vi "05 - Tip - Achieving Deterministic Handling Order.vi"() -> ()   [LabVIEW 2012]
panel:
  in  "Generate Events":enum16{"Greater than 1msec", "Sub-millisecond"}(ring)
  in  "Control":bool
  out "Static Event Registration":i32(graph)
  out "Dynamic Event Registration":i32(graph)
  out "Unique Event Queue":i32(graph)
  # "Conclusion:\nAll events within a single Events Queue will be handled deterministically;\nevents in separate Events Queues will be handled with millisecond accuracy,\nbut could become out of order with sub-millisecond resolution.\n\nBut don't count on handling order, especially near the 1msec threshold."
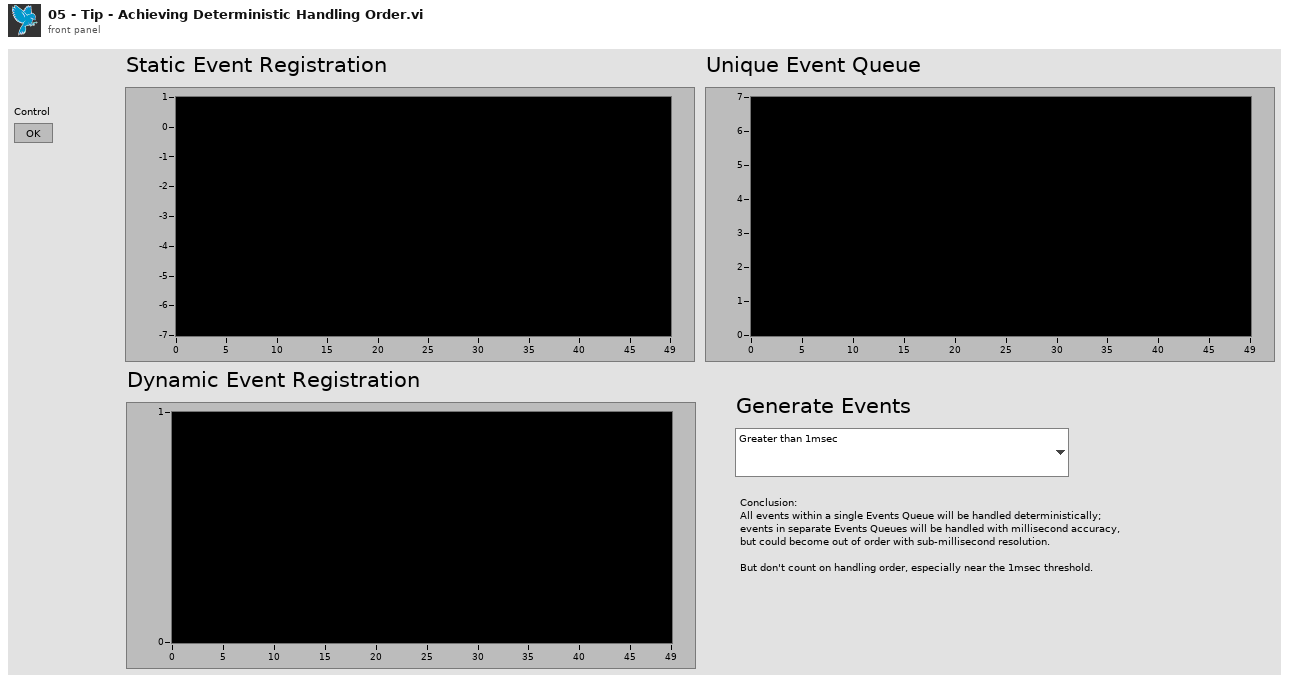
[diagram p1: front panel]
types:
  T1 = cluster{"Event Registration Refnum":refnum<event-registration>, "Event Registration Refnum":refnum<event-registration>}
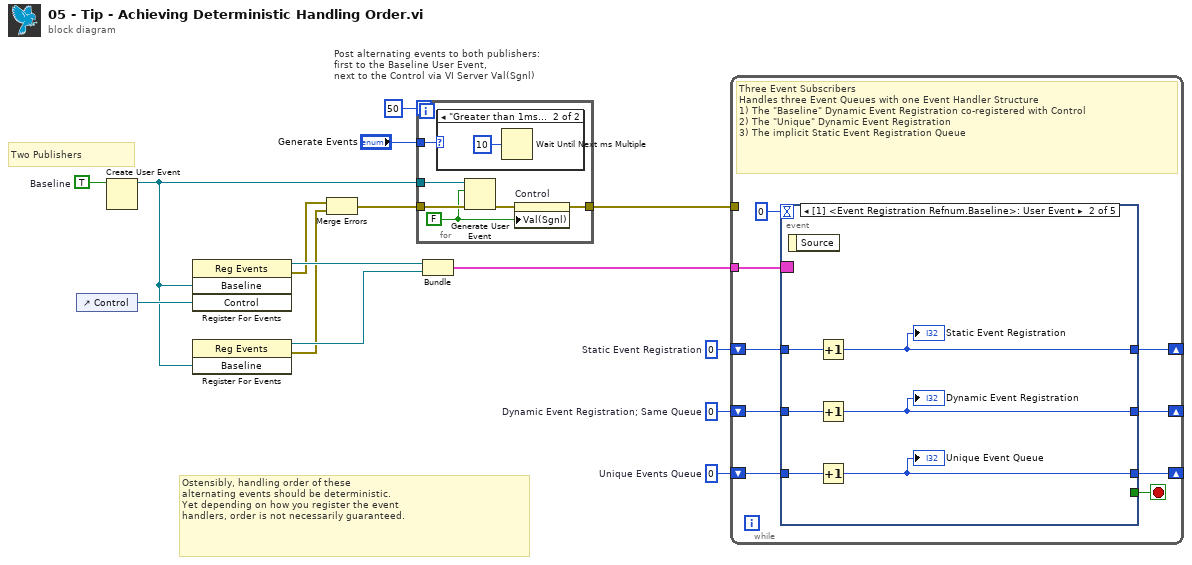
[diagram p0: block diagram]
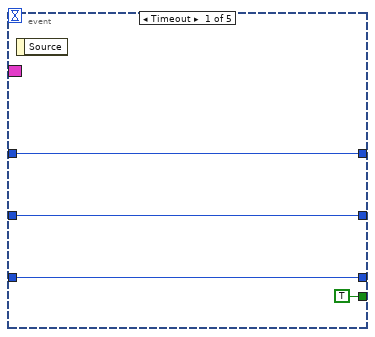
[diagram p3: hidden frame]
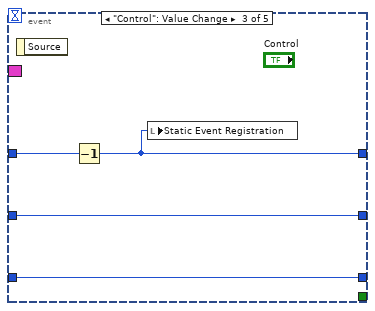
[diagram p4: hidden frame]
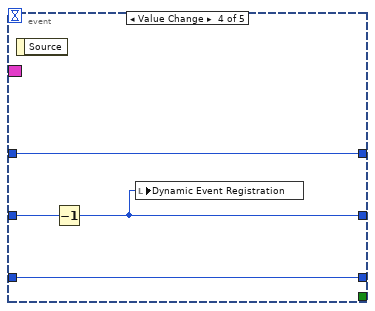
[diagram p5: hidden frame]
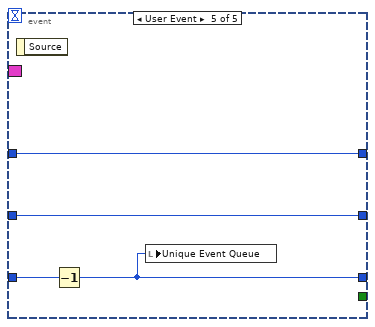
[diagram p6: hidden frame]
diagram:
  w5 = 0  # Unique Events Queue
  w10 = 0  # Dynamic Event Registration; Same Queue
  w12 = 0  # Static Event Registration
  w15 = TRUE  # Baseline
  # "Two Publishers"
  # "Ostensibly, handling order of these\nalternating events should be deterministic.\nYet depending on how you register the event\nhandlers, order is not necessarily guaranteed."
  n1 = control-ref of="Control"() -> (w11:refnum<vi>)
  n2 = Create User Event(user event datatype=w15) -> (user event=w9:refnum<user-event>)  [unwired: 1 in, 1 out]
  n3 = register-events(w9, w11) -> (reference out=w8:refnum<event-registration>, error out=w4:errorcluster)  [unwired: 2 in]
  n4 = register-events(w9) -> (reference out=w6:refnum<event-registration>, error out=w3:errorcluster)  [unwired: 2 in]
  n5 = Merge Errors(w4, w3) -> (w2:errorcluster)
  n6 = for "Post alternating events to both publishers:\nfirst to the Baseline User Event,\nnext to the Control via VI Server Val(Sgnl)" {
    N: 50 -> [_]
    tunnel: w9 -> [w20]
    tunnel: w2 -> [w19]
    tunnel: [w18] -> w13
    tunnel: "Generate Events" -> [w16]
    w17 = FALSE ("Value (Signaling)")
    n7 = case shown="\"Greater than 1msec\"" w16 {
      frame "Sub-millisecond" {
      }
      frame "Greater than 1msec" {
        n8 = Wait Until Next ms Multiple(millisecond multiple=u32 10 ("milliseconds to wait")) -> ()  [unwired: 1 out]
      }
    }
    n9 = Generate User Event(user event=w20, event data cluster=w17, error in=w19) -> (error out=w21:errorcluster)  [unwired: 1 out]
    n10 = property on="Control" class="Bool (strict)"(error in=w21, "Val(Sgnl)"=w17) -> (error out=w18:errorcluster)  [unwired: 1 in, 1 out]
  }
  n11 = Bundle("Event Registration Refnum"=w8, "Event Registration Refnum"=w6) -> (w7:T1)  [unwired: 1 in]
  n12 = while {
    tunnel: w7 -> [w31]
    tunnel: w13 -> [_]
    shift-right: [w27] -> _
    shift-left: w12 -> [w28]
    shift-right: [w25] -> _
    shift-left: w10 -> [w26]
    shift-right: [w24] -> _
    shift-left: w5 -> [w23]
    stop <- w30 stop-if-true
    # "Three Event Subscribers\nHandles three Event Queues with one Event Handler Structure\n1) The \"Baseline\" Dynamic Event Registration co-registered with Control\n2) The \"Unique\" Dynamic Event Registration\n3) The implicit Static Event Registration Queue"
    n13 = event shown="[1] <Event Registration Refnum.Baseline>: User Event" {
      selector: w31 -> [_ _ _ _ _]
      dyn-events: _ -> [_ _ _ _ _]
      timeout: 0 -> [_ _ _ _ _]
      tunnel: [TRUE _ _ _ _] -> w30
      tunnel: w28 -> [w34 w41 w45 w48 w53]
      tunnel: [w34 w36 w42 w48 w53] -> w27
      tunnel: w26 -> [w33 w40 w44 w49 w51]
      tunnel: [w33 w37 w44 w46 w51] -> w25
      tunnel: [w32 w38 w43 w47 w50] -> w24
      tunnel: w23 -> [w32 w39 w43 w47 w52]
      event Timeout {
        n14 = event-data() -> ()  [unwired: 1 in, 1 out]
      }
      event User Event {
        n15 = event-data() -> ()  [unwired: 1 in, 1 out]
        n16 = Increment(x=w41) -> (x+1=w36:i32)
        "Static Event Registration" <- w36
        n17 = Increment(x=w40) -> (x+1=w37:i32)
        "Dynamic Event Registration" <- w37
        n18 = Increment(x=w39) -> (x+1=w38:i32)
        "Unique Event Queue" <- w38
      }
      event "Control": Value Change {
        n19 = event-data() -> ()  [unwired: 1 in, 1 out]
        n20 = Decrement(x=w45) -> (x-1=w42:i32)
        n21 = local write "Static Event Registration"(w42) -> ()
      }
      event Value Change {
        n22 = event-data() -> ()  [unwired: 1 in, 1 out]
        n23 = Decrement(x=w49) -> (x-1=w46:i32)
        n24 = local write "Dynamic Event Registration"(w46) -> ()
      }
      event User Event {
        n25 = event-data() -> ()  [unwired: 1 in, 1 out]
        n26 = Decrement(x=w52) -> (x-1=w50:i32)
        n27 = local write "Unique Event Queue"(w50) -> ()
      }
    }
  }
